vi "CMD DoSomething.vi"(8 "error in (no error)":errorcluster, 11 "Database in":refnum<class "Database.lvclass">) -> (0 "error out":errorcluster, 3 "Database out":refnum<class "Database.lvclass">)   [LabVIEW 2022 SP3, in "Database.lvclass"]
doc: "Developed by Kevin Thompson\nkevin@thompsonengineering.net\n\nCopyright 2018\nThompson Engineering, LLC"
uses:
  Database.lvclass
  DataTypes/AsynCmd_Temp01--enum.ctl
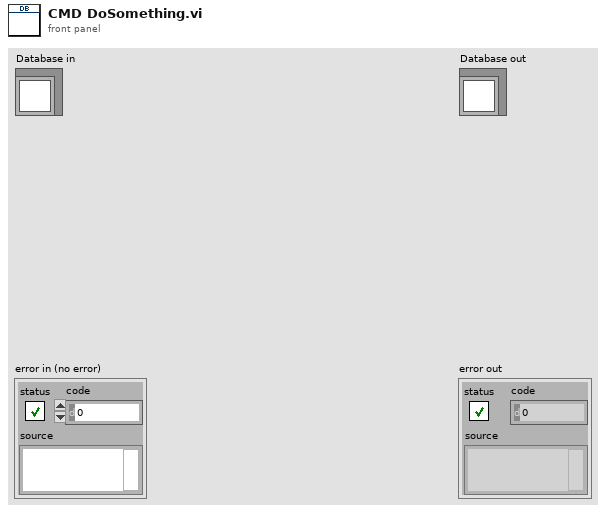
[diagram p1: front panel]
types:
  T1 = typedef "Database.lvclass/AsynCmd_Temp01--enum.ctl" = enum16{"DB.DeleteRecord", "DB.UpdateRecord", "DB.InsertRecord", "DB.SelectRecord", "DB.ExecuteSQLCommand", "DB.FindFirstSlot", "DB.GenericSQLQuery"}
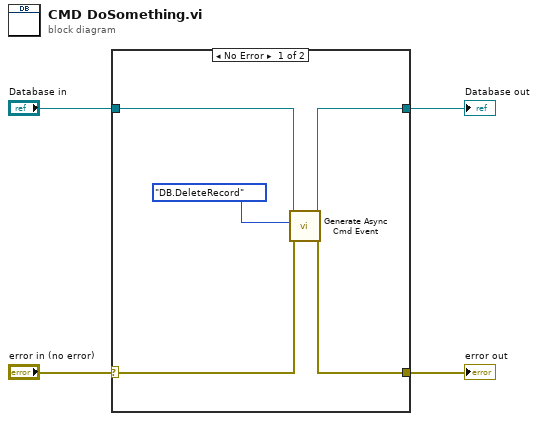
[diagram p0: block diagram]
diagram:
  n1 = case shown="No Error" "error in (no error)" {
    selector: "error in (no error)" -> [w7 w11]
    tunnel: [w6 w11] -> w3
    tunnel: [w8 w10] -> w1
    tunnel: "Database in" -> [w9 w10]
    frame No Error {
      n2 = call "Generate Async Cmd Event.vi"("error in (no error)"=w7, "AsyncCmd"=AsynCmd_Temp01--enum."DB.DeleteRecord", "Database in"=w9) -> ("error out"=w6:errorcluster, "Database out"=w8:refnum<class "Database.lvclass">)  [unwired: 7 in]
    }
    frame Error {
    }
  }
  "error out" <- w3
  "Database out" <- w1
